vi "All off Except.vi"(8 "error in (no error)":errorcluster, 10 "Numeric":u8 max=20, 11 "VISA resource name":refnum<visa-resource-name>) -> (0 "error out":errorcluster, 1 "read buffer":string, 2 "All sent strings":string[](array[string]), 3 "VISA resource name out":refnum<visa-resource-name>)   [LabVIEW 2012, in "Fluke 2625A.lvlib"]
uses:
  <instrlib>/Fluke 2625A/Fluke 2625A.lvlib
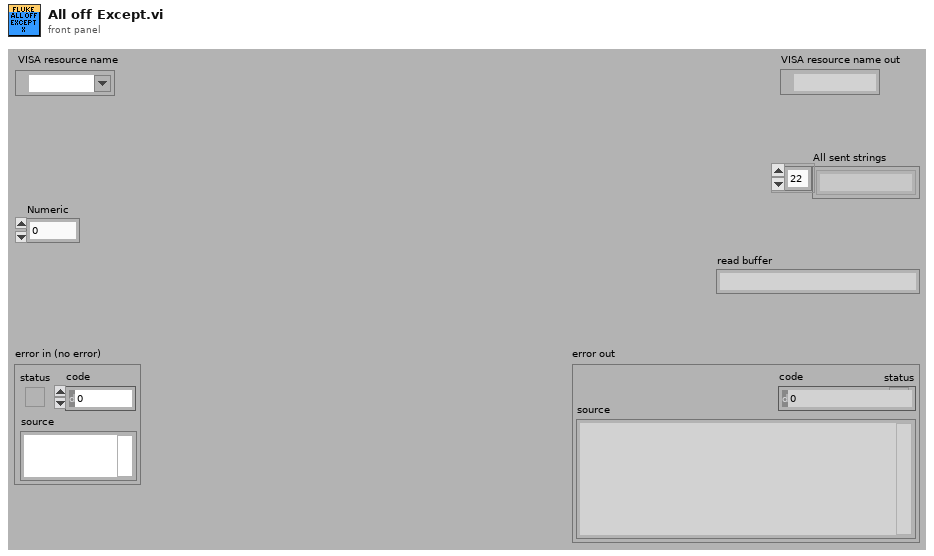
[diagram p1: front panel]
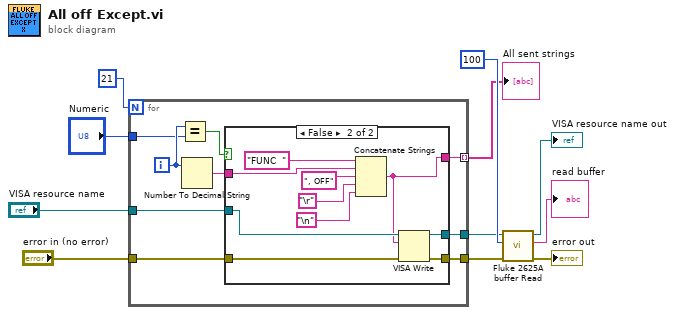
[diagram p0: block diagram]
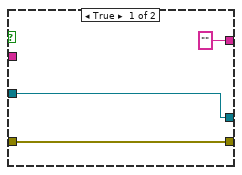
[diagram p2: hidden frame]
diagram:
  n1 = for {
    N: 21 -> [_]
    tunnel: [w20] -> w7
    tunnel: [w19] -> w6
    tunnel: "VISA resource name" -> [w17]
    tunnel: "error in (no error)" -> [w16]
    tunnel: [w15] -> w2 mode=indexing
    tunnel: "Numeric" -> [w12]
    i -> [w13]
    n2 = Equal?(x=w13, y=w12) -> (x = y?=w14:bool)
    n3 = Number To Decimal String(number=w13) -> (decimal integer string=w18:string)  [unwired: 1 in]
    n4 = case shown="False" w14 {
      tunnel: [w21 w33] -> w20
      tunnel: [w22 w32] -> w19
      tunnel: w18 -> [_ w30]
      tunnel: w17 -> [w22 w29]
      tunnel: w16 -> [w21 w28]
      tunnel: ["" w27] -> w15
      frame True {
      }
      frame False {
        n5 = Concatenate Strings("FUNC  " ("string"), w30, ", OFF" ("string"), "\r", "\n") -> (w27:string)
        n6 = VISA Write(VISA resource name=w29, write buffer=w27, error in (no error)=w28) -> (VISA resource name out=w32:refnum<visa-resource-name>, error out=w33:errorcluster)  [unwired: 1 out]
      }
    }
  }
  "All sent strings" <- w2
  n7 = call <instrlib>:"Fluke 2625A buffer Read.vi"("error out"=w7, "byte count"=u32 100, "VISA resource name out"=w6) -> ("error out 2"=→"error out":errorcluster, "read buffer"=→"read buffer":string, "VISA resource name out 2"=→"VISA resource name out":refnum<visa-resource-name>)  [unwired: 5 in, 1 out]
